vi "import.vi"() -> ()   [LabVIEW 2020]
uses:
  <vilib>/Utility/file.llb/Read Delimited Spreadsheet (string).vi
  <vilib>/Utility/file.llb/Read Delimited Spreadsheet (DBL).vi
panel:
  out "position on sky":picture
  in  "stop":bool
  out "Altitude and Azimuth Of Object":string
  out "Object And Location":string
  out "Latitude":dbl
  out "Longitude":dbl
  in  "Body":u16(ring) items=["Sun", "Moon", "Mercury", "Venus", "Mars", "Phobos", "Deimos", "Jupiter", "Io", "Europa", "Ganymede", "Calisto", "Saturn", "Uranus", "Neptune", "Pluto", "Sirrah", "Caph", "Algenib", "Schedar", "Mirach", "Achernar", "Almach", "Hamal", "Polaris", "Menkar", "Algol", "Electra", "Taygeta", "Maia", "Merope", "Alcyone", "Atlas", "Zaurak", "Aldebaran", "Rigel", "Capella", "Bellatrix", "Elnath", "Nihal", "Mintaka", "Arneb", "Alnilam", "Alnitak", "Saiph", "Betelgeuse", "Menkalinan", "Mirzam", "Canopus", "Alhena", "Sirius", "Adara", "Wezen", "Castor", "Procyon", "Pollux", "Naos", "Alphard", "Regulus", "Algieba", "Merak", "Dubhe", "Denebola", "Phecda", "Minkar", "Megrez", "Gienah Corvi", "Mimosa", "Alioth", "Vindemiatrix", "Mizar", "Spica", "Alcor", "Alcaid", "Agena", "Thuban", "Arcturus", "Izar", "Kochab", "Alphecca", "Unukalhai", "Antares", "Rasalgethi", "Shaula", "Rasalhague", "Cebalrai", "Etamin", "Kaus Australis", "Vega", "Sheliak", "Nunki", "Sulafat", "Arkab Prior", "Arkab Posterior", "Rukbat", "Albereo", "Tarazed", "Altair", "Alshain", "Sadr", "Peacock", "Deneb", "Alderamin", "Alfirk", "Enif", "Sadalmelik", "Alnair", "Fomalhaut", "Scheat", "Markab", "Acamar", "Acrux", "Adhara", "Alkaid", "Alpheratz", "Ankaa", "Atria", "Avior", "Diphda", "Eltanin", "Formalhaut", "Gacrux", "Gienah", "Hadar", "Menkent", "Miaplacidus", "Mirfak", "Rigil Kentaurus", "Sabik", "Suhail", "Zubenelgenubi"]
  in  "City":u16(ring) items=["city", "‘Abbasabad", "‘Ajab Shir", "‘Aliabad-e Katul", "‘Anbarabad", "Ab Bar", "Abadan", "Abadeh", "Abarkuh", "Abdanan", "Abhar", "Abu Musa", "Abyek", "Ahar", "Ahram", "Ahvaz", "Aleshtar", "Aligudarz", "Alvand", "Amlash", "Amol", "Anar", "Andimeshk", "Aq Qala", "Aradan", "Arak", "Arakvaz-e Malekshahi", "Aran Bidgol", "Ardabil", "Ardakan", "Ardal", "Ardestan", "Ardsalem", "Arsanjan", "Arzu’iyeh", "Asadabad", "Asadiyeh", "Ashkez¯ar", "Ashkhaneh", "Ashtian", "Astaneh-ye Ashrafiyeh", "Astara", "Azadshahr", "Az¯arshahr", "Azna", "Babol", "Babolsar", "Bafq", "Baft", "Bagh-e Malek", "Bahar", "Bajestan", "Bam", "Bandar ‘Abbas", "Bandar-e ‘Asaluyeh", "Bandar-e Anzali", "Bandar-e Bushehr", "Bandar-e Deylam", "Bandar-e Ganaveh", "Bandar-e Gaz", "Bandar-e Khamir", "Bandar-e Lengeh", "Bandar-e Mahshahr", "Bandar-e Torkaman", "Baneh", "Bardaskan", "Bardsir", "Basht", "Bastak", "Behabad", "Behbahan", "Behshahr", "Bijar", "Bileh Savar", "Birjand", "Bojnurd", "Bonab", "Borazjan", "Borujen", "Borujerd", "Boshruyeh", "Bostanabad", "Bozghan", "Bu’in Zahra", "Bukan", "Chabahar", "Chadegan", "Chalus", "Charam", "Chelgard", "Chenaran", "Dalgan", "Damavand", "Damghan", "Darab", "Daran", "Dargaz", "Darreh Shahr", "Dehaqan", "Dehdasht", "Dehgolan", "Dehloran", "Delijan", "Deyr", "Dezful", "Divandarreh", "Do Gonbadan", "Dorud", "Dowlatabad", "Dowlatabad", "Dust Mo?ammad Khan", "Eqlid", "Esfahan", "Esfarayen", "Eshtehard", "Eslamabad", "Eslamabad-e Gharb", "Eslamshahr", "Estahban", "Eyvan", "Fahraj", "Falavarjan", "Famenin", "Farashband", "Fareydunshahr", "Fariman", "Farmahin", "Farsan", "Faruj", "Faryab", "Fasa", "Ferdows", "Fereydunkenar", "Fey?abad", "Firuzabad", "Firuzkuh", "Fuman", "Galikesh", "Galugah", "Garmeh", "Garmsar", "Gavbandi", "Gerash", "Germi", "Gilan-e Gharb", "Givi", "Golpayegan", "Gomishan", "Gonabad", "Gonbad-e Kavus", "Gorgan", "Haftkel", "?ajjiabad", "?ajjiabad", "?ajjiabad", "Hamadan", "Harsin", "Hashtgerd", "Hashtpar", "Hashtrud", "Hendijan", "Heris", "Hoveyzeh", "Ilam", "Iranshahr", "Iz¯eh", "Jahrom", "Jajarm", "Jam", "Jask", "Javanrud", "Jiroft", "Joghtay", "Jolfa", "Juybar", "Kabudarahang", "Kahnuj", "Kalaleh", "Kalat-e Naderi", "Kaleybar", "Kamyaran", "Kangan", "Kangavar", "Karaj", "Kashan", "Kashmar", "Kavar", "Kazerun", "Kerend-e Gharb", "Kerman", "Kermanshah", "Khalilabad", "Khalkhal", "Khash", "Kherameh", "Khodabandeh", "Khomarlu", "Khomeyn", "Khomeyni Shahr", "Khondab", "Khonj", "Khorramabad", "Khorramdarreh", "Khorramshahr", "Khowrmuj", "Khur", "Khvaf", "Khvansar", "Khvoy", "Komijan", "Konarak", "Kord Kuy", "Kuhbanan", "Kuhdasht", "Lahijan", "Lali", "Lamerd", "Langarud", "Likak", "Lordegan", "Mahabad", "Ma?allat", "Ma?mudabad", "Mahneshan", "Maku", "Malard", "Malayer", "Malekan", "Mamuniyeh", "Manujan", "Maragheh", "Marand", "Maraveh Tappeh", "Marivan", "Marvdasht", "Masal", "Mashhad", "Masiri", "Masjed Soleyman", "Mehdishahr", "Mehran", "Mehriz", "Meshgin Shahr", "Meyami", "Meybod", "Miandoab", "Mianeh", "Minab", "Minudasht", "Mobarakeh", "Mo?ammadabad", "Mohr", "Mollas¯ani", "Na’in", "Nahavand", "Najafabad", "Namin", "Naqadeh", "Narmashir", "Nasim Shahr", "Natanz", "Naz¸arabad", "Nehbandan", "Neka", "Neqab", "Neyriz", "Nikshahr", "Nir", "Nishabur", "Nowshahr", "Nur", "Nurabad", "Nurabad", "Omidiyeh", "Orumiyeh", "Oshnaviyeh", "Osku", "Pa’in-e Bazar-e Rudbar", "Pakdasht", "Parsabad", "Paveh", "Piranshahr", "Pishva", "Poldasht", "Poldokhtar", "Pol-e Sefid", "Qa’em Shahr", "Qa’en", "Qal‘eh Ganj", "Qal‘eh-ye Khvajeh", "Qarah Aghaj", "Qarah ?ia’ od Din", "Qasr-e Shirin", "Qazvin", "Qeshm", "Qir", "Qom", "Qorveh", "Quchan", "Rabor", "Rafsanjan", "Ramhormoz", "Ramian", "Ramsar", "Ramshir", "Rasak", "Rasht", "Ravansar", "Ravar", "Razan", "Rey", "Re?vanshahr", "Robat Karim", "Roshtkhvar", "Rudan", "Rudsar", "Sa‘adat Shahr", "Sabzevar", "Safashahr", "Sa?neh", "Salmas", "Sanandaj", "Saqqez", "Sar‘eyn", "Sarab", "Sarab-e Dowreh", "Sarableh", "Sarakhs", "Sarayan", "Sarbisheh", "Sardasht", "Sardasht", "Sari", "Sarpol-e Z¯ahab", "Sarvabad", "Sarvestan", "Saveh", "Semirom", "Semnan", "Sepidan", "Seyah Cheshmeh", "Shabestar", "Shadegan", "Shaft", "Shahin Dezh", "Shahin Shahr", "Shahrak-e Bakharz", "Shahr-e Babak", "Shahr-e Herat", "Shahr-e Kord", "Shahr-e Qadim-e Lar", "Shahr-e Qods", "Shahre?a", "Shahriar", "Shahrud", "Shalamzar", "Shazand", "Shiraz", "Shirvan", "Showt", "Shush", "Shushtar", "Siahkal", "Sirik", "Sirjan", "Sisakht", "Soltanabad", "Sonqor", "Sorkheh", "Sowme‘eh Sara", "Surak", "Suran", "Surian", "Susangerd", "Tabas", "Tabriz", "Tafresh", "Taft", "Tajrish", "Takab", "Takestan", "Taleqan", "Taybad", "Tazehabad", "Tehran", "Tiran", "Tonekabon", "Torbat-e ?eydariyeh", "Torbat-e Jam", "Torqabeh", "Tuyserkan", "Varamin", "Varazqan", "Yasuj", "Yazd", "Zabol", "Zaboli", "Zahedan", "Zanjan", "Zarand", "Zarrin Shahr", "Zarrinabad", "Zehak"]
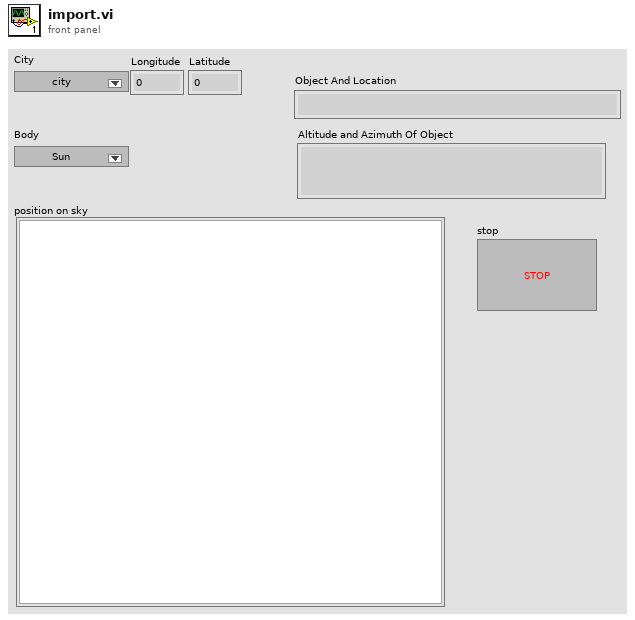
[diagram p1: front panel]
types:
  T1 = cluster{"maximum":dbl, "minimum":dbl, "clip to min":bool, "log?(F)":bool, "grid color":u32, "plot color":u32, "fmt and prec":cluster{"format":enum8{"Decimal", "Scientific", "Engineering", "Binary", "Octal", "Hex"}, "precision":u8}, "visible section":u16}
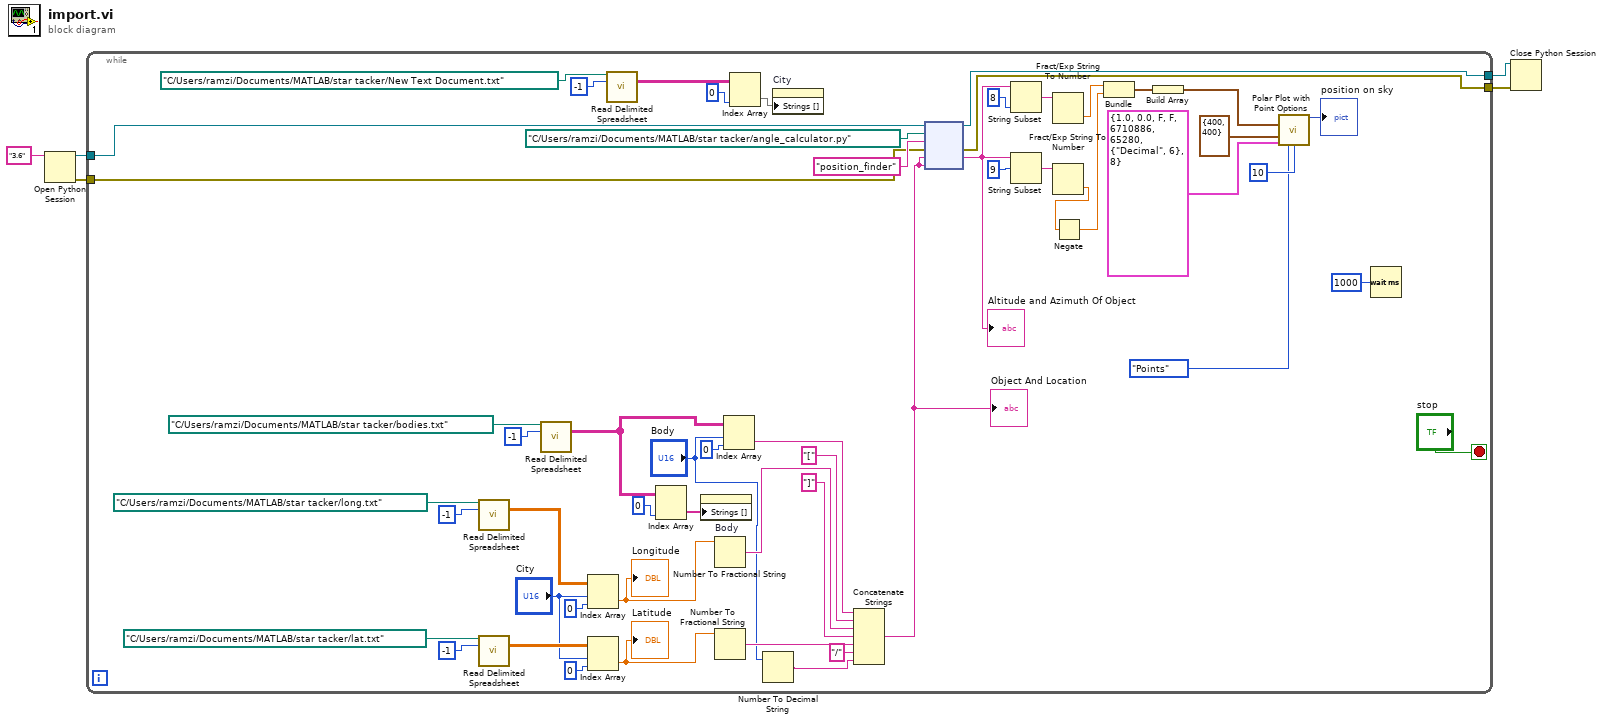
[diagram p0: block diagram]
diagram:
  n1 = Open Python Session(python version="3.6" ("Python version")) -> (session out=w4:refnum<k35>, error out=w3:errorcluster)  [unwired: 2 in]
  n2 = while {
    tunnel: w4 -> [w32]
    tunnel: w3 -> [w11]
    tunnel: [w30] -> w2
    tunnel: [w29] -> w1
    stop <- "stop" stop-if-true
    n3 = call-poly <vilib>:"Read Delimited Spreadsheet.vi"("file path (dialog if empty)"=path "C:/Users/ramzi/Documents/MATLAB/star tacker/long.txt", "number of rows (all:-1)"=-1) -> ("all rows"=w49:dbl[][])  [unwired: 8 in, 5 out]
    n4 = call-poly <vilib>:"Read Delimited Spreadsheet.vi"("file path (dialog if empty)"=path "C:/Users/ramzi/Documents/MATLAB/star tacker/lat.txt", "number of rows (all:-1)"=-1) -> ("all rows"=w53:dbl[][])  [unwired: 8 in, 5 out]
    n5 = call-poly <vilib>:"Read Delimited Spreadsheet.vi"("file path (dialog if empty)"=path "C:/Users/ramzi/Documents/MATLAB/star tacker/bodies.txt", "number of rows (all:-1)"=-1) -> ("all rows"=w12:string[][])  [unwired: 8 in, 5 out]
    n6 = Index Array(array=w49, index (row)="City", index (col)=0 ("disabled index (col)")) -> (element=w34:dbl)
    "Longitude" <- w34
    n7 = Index Array(array=w53, index (row)="City", index (col)=0 ("disabled index (col)")) -> (element=w33:dbl)
    "Latitude" <- w33
    n8 = call-poly <vilib>:"Read Delimited Spreadsheet.vi"("file path (dialog if empty)"=path "C:/Users/ramzi/Documents/MATLAB/star tacker/New Text Document.txt", "number of rows (all:-1)"=-1) -> ("all rows"=w58:string[][])  [unwired: 8 in, 5 out]
    n9 = Index Array(array=w12, index (col)=0 ("disabled index (col)")) -> (element=w43:string[])  [unwired: 1 in]
    n10 = property on="Body" class="Ring (strict)"("Strings []"=w43) -> ()  [unwired: 2 in, 2 out]
    n11 = Number To Fractional String(number=w34) -> (F-format string=w36:string)  [unwired: 3 in]
    n12 = Number To Fractional String(number=w33) -> (F-format string=w37:string)  [unwired: 3 in]
    n13 = Index Array(array=w12, index (row)="Body", index (col)=0 ("disabled index (col)")) -> (element=w40:string)
    n14 = Index Array(array=w58, index (col)=0 ("disabled index (col)")) -> (element=w56:string[])  [unwired: 1 in]
    n15 = Number To Decimal String(number="Body") -> (decimal integer string=w9:string)  [unwired: 1 in]
    n16 = property on="City" class="Ring (strict)"("Strings []"=w56) -> ()  [unwired: 2 in, 2 out]
    n17 = Concatenate Strings(w40, "[" ("string"), w36, "]" ("string"), w37, "/" ("string"), w9) -> (w10:string)
    "Object And Location" <- w10
    n18 = node(w32, path "C:/Users/ramzi/Documents/MATLAB/star tacker/angle_calculator.py" ("Path to Python Module (.py File)"), "position_finder" ("function name"), w11, w10, w10) -> (w30:refnum<k35>, w29:errorcluster, w24:string)  [unwired: 1 in, 2 out]
    "Altitude and Azimuth Of Object" <- w24
    n19 = String Subset(string=w24, length (rest)=8 ("length (rest)")) -> (substring=w21:string)  [unwired: 1 in]
    n20 = String Subset(string=w24, offset (0)=9) -> (substring=w20:string)  [unwired: 1 in]
    n21 = Fract/Exp String To Number(string=w21) -> (number=w17:dbl)  [unwired: 3 in, 1 out]
    n22 = Fract/Exp String To Number(string=w20) -> (number=w7:dbl)  [unwired: 3 in, 1 out]
    n23 = Negate(x=w7) -> (-x=w6:dbl)
    n24 = Bundle(w17, w6) -> (w19:cluster{dbl, dbl})  [unwired: 1 in]
    n25 = Build Array(w19) -> (w18:cluster{dbl, dbl}[])
    n26 = call <vilib>:"Polar Plot with Point Options.vi"("data array [mag, phase (deg)]"=w18, "dimensions (w,h)"=cluster{"width":i16, "height":i16} {"width"=400, "height"=400}, "polar attributes"=T1 {"maximum"=1.0, "minimum"=0.0, "clip to min"=FALSE, "log?(F)"=FALSE, "grid color"=6710886, "plot color"=65280, "fmt and prec"={"format"=enum."Decimal", "precision"=6}, "visible section"=8}, "Lines/Points"=enum16{"Lines", "Points"}."Points", "Size"=u16 10) -> ("new picture"=→"position on sky":picture)  [unwired: 10 in]
    n27 = Wait (ms)(milliseconds to wait=u32 1000) -> ()  [unwired: 1 out]
  }
  n28 = Close Python Session(session in=w2, error in=w1) -> ()  [unwired: 1 out]
